vi "Get Default Step Settings.vi"(10 "Num of Digital Channels":i32, 11 "Num of Analog Channels":i32) -> (3 "Default Step Settings":T1)   [LabVIEW 2020, in "Sequencer with Output Values.lvlib" / "Sequencer with Output Values.lvclass"]
uses:
  Sequencer with Output Values.lvclass
  Step Settings.ctl
  Global Strings.vi
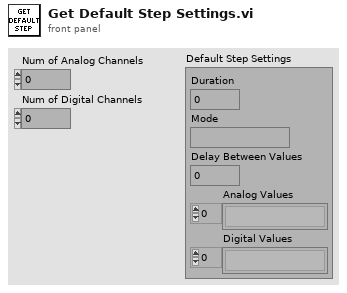
[diagram p1: front panel]
types:
  T1 = typedef "Sequencer with Output Values.lvlib/Sequencer with Output Values.lvclass/Step Settings.ctl" = cluster{"Duration":dbl, "Mode":string, "Delay Between Values":dbl, "Analog Values":string[], "Digital Values":string[]}
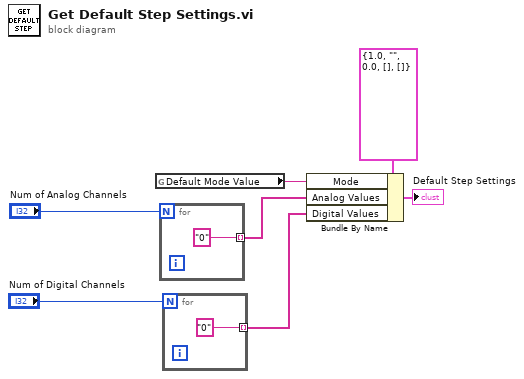
[diagram p0: block diagram]
diagram:
  n1 = global read "Global Strings.vi" "Default Mode Value"() -> (w6:string)
  n2 = for {
    N: "Num of Analog Channels" -> [_]
    tunnel: ["0"] -> w4 mode=indexing
  }
  n3 = for {
    N: "Num of Digital Channels" -> [_]
    tunnel: ["0"] -> w2 mode=indexing
  }
  n4 = Bundle By Name(cluster=T1 {"Duration"=1.0, "Mode"="", "Delay Between Values"=0.0, "Analog Values"=[], "Digital Values"=[]} ("Step Settings"), "Mode"=w6, "Analog Values"=w4, "Digital Values"=w2) -> (→"Default Step Settings":T1)
